vi "Adjust lib ICON.vi"(6 "Debug":bool, 8 "error in":errorcluster, 10 "Overlay Icon":refnum<class "Icon.lvclass">, 11 "Name to Lib Map":map{string, refnum<vi>}(c390)) -> (0 "error out":errorcluster caption="error in", 3 "Name to Lib Map out":map{string, refnum<vi>}(c390), 4 "Result for debugging":cluster{"Name":string, picture[]}[](array[cluster]))   [LabVIEW 2023, in "Plugin Generator.lvlib"]
uses:
  Plugin Generator.lvlib
  <vilib>/LabVIEW Icon API/lv_icon/Classes/Icon/Icon.lvclass
  <vilib>/LabVIEW Icon API/Support/Get Data from Icon Class.vi
  <vilib>/LabVIEW Icon API/lv_icon/Classes/Layer/Substitute Layer.vi
  <vilib>/LabVIEW Icon API/Support/Get Icon Class from Data.vi
  <vilib>/LabVIEW Icon API/Set VI Icon.vi
  <vilib>/LabVIEW Icon API/LabVIEW Icon API.lvlib
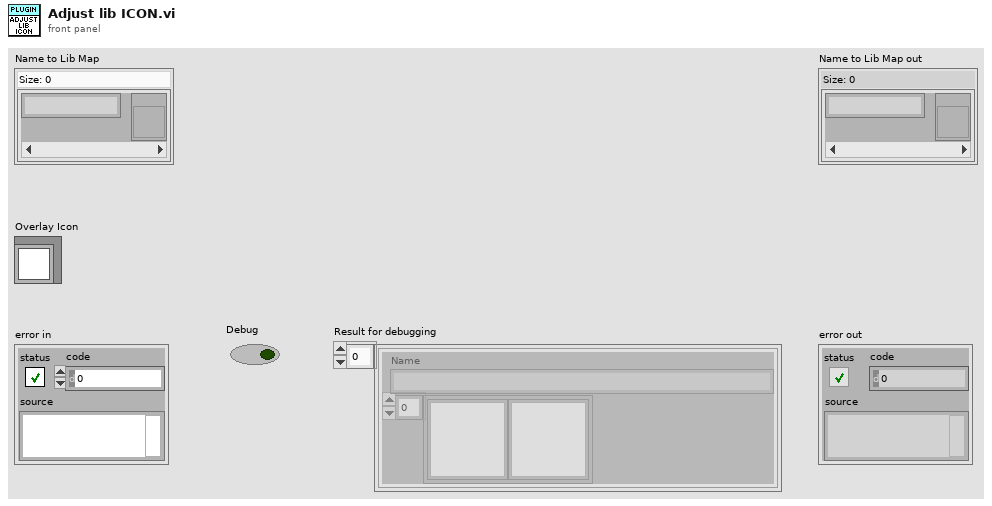
[diagram p1: front panel]
types:
  T1 = typedef "imagedata.ctl" = cluster{"image type":i32, "image depth":i32, "image":u8[], "mask":u8[], "colors":u32[], "Rectangle":cluster{"left":i16, "top":i16, "right":i16, "bottom":i16}}
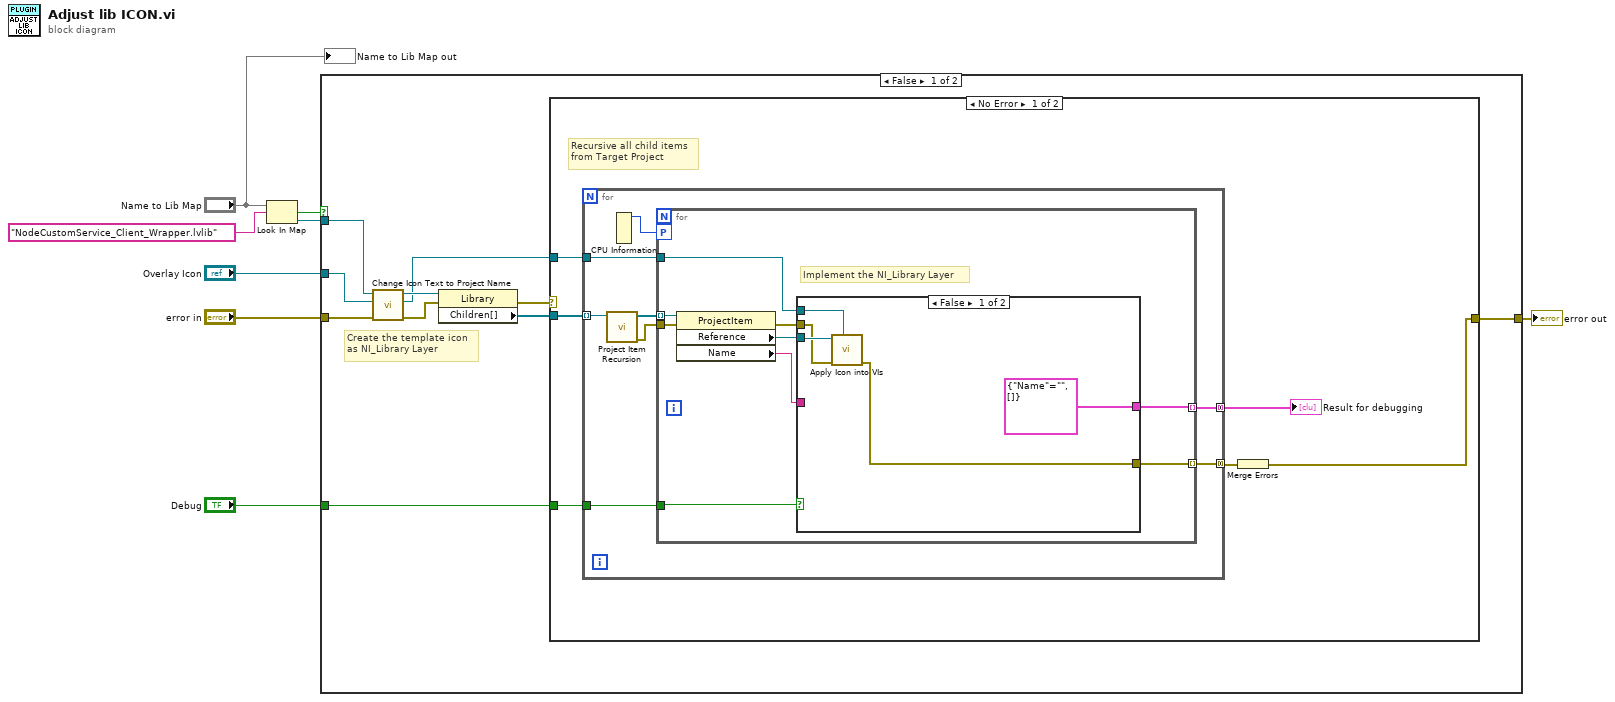
[diagram p0: block diagram]
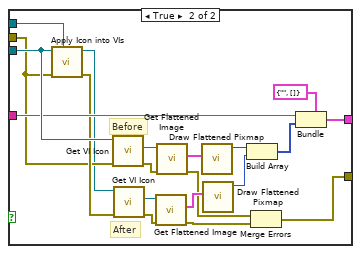
[diagram p2: hidden frame]
diagram:
  n1 = Look In Map(map="Name to Lib Map", key="NodeCustomService_Client_Wrapper.lvlib" ("String")) -> (key not found?=w6:bool, value=w5:refnum<vi>)  [unwired: 1 in]
  n2 = case shown="False" w6 {
    tunnel: w5 -> [w17 _]
    tunnel: "Debug" -> [w14 _]
    tunnel: "error in" -> [w13 w68]
    tunnel: [w12 w68] -> w2
    tunnel: "Overlay Icon" -> [w9 _]
    frame False {
      # "Create the template icon\nas NI_Library Layer"
      n3 = call "Change Icon Text to Project Name.vi"("error in"=w13, "Overlay Icon"=w9, "Lvclass Ref in"=w17) -> ("error out"=w16:errorcluster, "Layer.lvclass out"=w10:refnum<class "Layer.lvclass">, "Lvclass Ref out"=w11:refnum<vi>)  [unwired: 5 in, 1 out]
      n4 = property class="Library"(reference=w11, error in=w16) -> (error out=w15:errorcluster, "Children[]"=w18:refnum<vi>[])  [unwired: 1 out]
      n5 = case shown="No Error" w15 {
        selector: w15 -> [_ w67]
        tunnel: w18 -> [w24 _]
        tunnel: w10 -> [w22 _]
        tunnel: w14 -> [w21 _]
        tunnel: [w19 w67] -> w12
        frame No Error {
          # "Recursive all child items\nfrom Target Project"
          n6 = for {
            tunnel: w24 -> [w32] mode=indexing
            tunnel: [w30] -> w23 mode=concatenating
            tunnel: w22 -> [w28]
            tunnel: w21 -> [w26]
            tunnel: [w25] -> w20 mode=concatenating
            n7 = call "Project Item Recursion.vi"("TargetItem in"=w32) -> ("error out"=w29:errorcluster, "TargetItem out"=w31:refnum<vi>[])  [unwired: 9 in]
            n8 = CPU Information() -> (4:w27:i32)  [unwired: 3 out]
            n9 = for {
              tunnel: w31 -> [w41] mode=indexing
              tunnel: w29 -> [w40]
              tunnel: [w39] -> w30 mode=indexing
              tunnel: w28 -> [w33]
              workers-P: w27 -> [_]
              tunnel: w26 -> [w34]
              tunnel: [w36] -> w25 mode=indexing
              # "Implement the NI_Library Layer"
              n10 = property class="ProjectItem"(reference=w41, error in=w40) -> (error out=w35:errorcluster, "Reference"=w38:refnum<vi>, "Name"=w37:string)  [unwired: 1 out]
              n11 = case shown="False" w34 {
                tunnel: [cluster{"Name":string, picture[]} {"Name"="", []} ("cluster") w66] -> w39
                tunnel: w38 -> [w46 w65]
                tunnel: w37 -> [_ w64]
                tunnel: [w43 w62] -> w36
                tunnel: w35 -> [w45 w49]
                tunnel: w33 -> [w44 w48]
                frame False {
                  n12 = call "Apply Icon into VIs.vi"("Substitute Layer"=w44, "error in"=w45, "VI in"=w46) -> ("error out"=w43:errorcluster)  [unwired: 7 in, 1 out]
                }
                frame True {
                  # "After"
                  # "Before"
                  n13 = call "Apply Icon into VIs.vi"("Substitute Layer"=w48, "error in"=w49, "VI in"=w65) -> ("error out"=w63:errorcluster, "VI Refnum out"=w47:refnum<vi>)  [unwired: 7 in]
                  n14 = call <vilib>:"Get VI Icon.vi"("error in (no error)"=w49, "VI Refnum in"=w65) -> ("error out"=w53:errorcluster, "Icon"=w59:refnum<class "Icon.lvclass">)  [unwired: 7 in, 1 out]
                  n15 = call <vilib>:"Get VI Icon.vi"("error in (no error)"=w63, "VI Refnum in"=w47) -> ("error out"=w52:errorcluster, "Icon"=w61:refnum<class "Icon.lvclass">)  [unwired: 7 in, 1 out]
                  n16 = call <vilib>:"Get Flattened Image.vi"("error in (no error)"=w52, "lv_icon.lvlib:Icon.lvclass in"=w61) -> ("error out"=w50:errorcluster, "Color Image"=w60:T1)  [unwired: 6 in, 2 out]
                  n17 = call <vilib>:"Get Flattened Image.vi"("error in (no error)"=w53, "lv_icon.lvlib:Icon.lvclass in"=w59) -> ("error out"=w51:errorcluster, "Color Image"=w58:T1)  [unwired: 6 in, 2 out]
                  n18 = call <vilib>:"Draw Flattened Pixmap.vi"("image data"=w58) -> ("new picture"=w57:picture)  [unwired: 8 in]
                  n19 = call <vilib>:"Draw Flattened Pixmap.vi"("image data"=w60) -> ("new picture"=w56:picture)  [unwired: 8 in]
                  n20 = Build Array(w57, w56) -> (w55:picture[])
                  n21 = Merge Errors(w51, w50) -> (w62:errorcluster)
                  n22 = Bundle(cluster=cluster{"Name":string, picture[]} {"Name"="", []}, "Name"=w64, w55) -> (w66:cluster{"Name":string, picture[]})
                }
              }
            }
          }
          "Result for debugging" <- w23
          n23 = Merge Errors(w20) -> (w19:errorcluster)
        }
        frame Error {
        }
      }
    }
    frame True {
    }
  }
  "error out" <- w2
  "Name to Lib Map out" <- "Name to Lib Map"
